vi "VerifConnection.vi"(8 "error in (no error)":errorcluster, 9 "timeout in ms (1000)":u32=1000, 10 "device connected in":bool, 11 "Server in":refnum<class "Server.lvclass">) -> (0 "error out":errorcluster, 3 "Server out":refnum<class "Server.lvclass">)   [LabVIEW 2018, in "Server.lvclass"]
uses:
  Server.lvclass
  Server.lvclass/Server.ctl
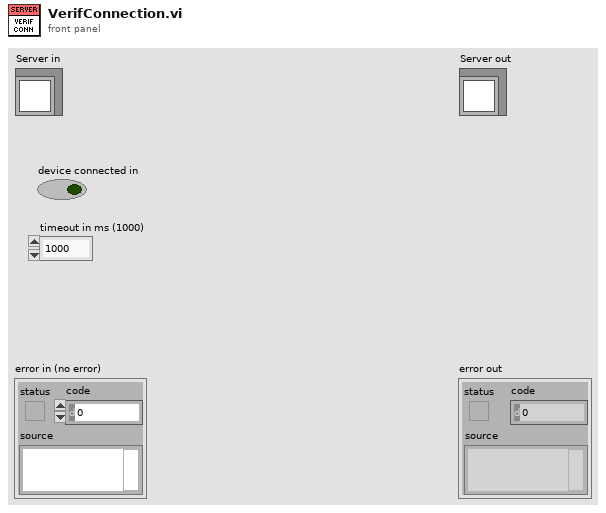
[diagram p1: front panel]
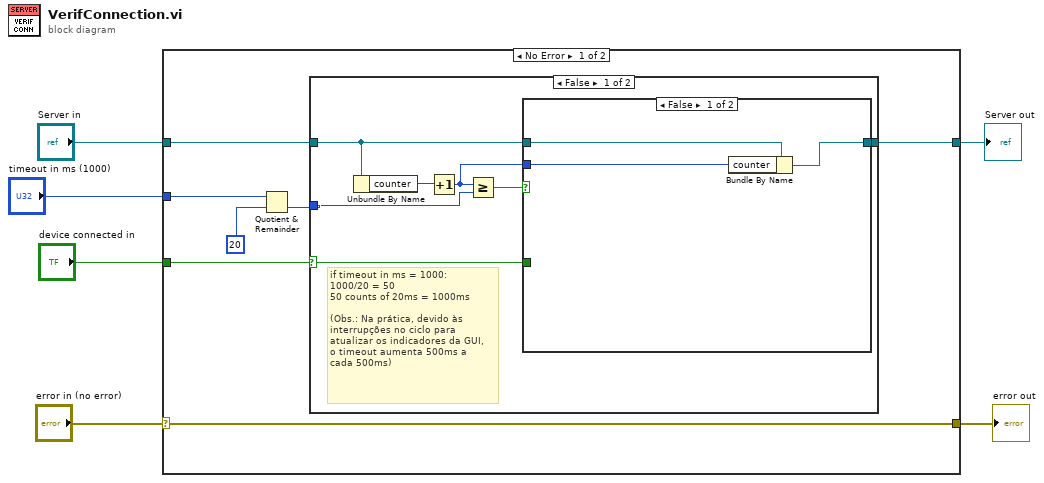
[diagram p0: block diagram]
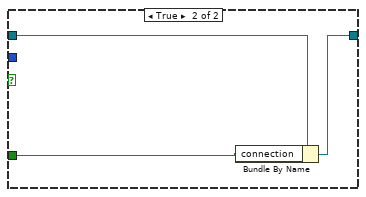
[diagram p2: hidden frame]
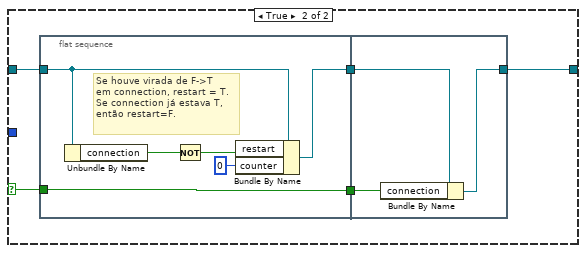
[diagram p3: hidden frame]
diagram:
  n1 = case shown="No Error" "error in (no error)" {
    selector: "error in (no error)" -> [w10 w42]
    tunnel: [w10 w42] -> w5
    tunnel: [w11 w41] -> w3
    tunnel: "Server in" -> [w13 w41]
    tunnel: "device connected in" -> [w12 _]
    tunnel: "timeout in ms (1000)" -> [w9 _]
    frame No Error {
      n2 = Quotient & Remainder(x=w9, y=u32 20) -> (floor(x/y)=w7:u32)  [unwired: 1 out]
      n3 = case shown="False" w12 {
        selector: w12 -> [w17 w29]
        tunnel: w13 -> [w19 w31]
        tunnel: [w16 w27] -> w11
        tunnel: w7 -> [w14 _]
        frame False {
          # "if timeout in ms = 1000:\n1000/20 = 50\n50 counts of 20ms = 1000ms\n\n(Obs.: Na prática, devido às\ninterrupções no ciclo para \natualizar os indicadores da GUI, \no timeout aumenta 500ms a \ncada 500ms)"
          n4 = Unbundle By Name(w19) -> ("counter"=w20:u32)
          n5 = Increment(x=w20) -> (x+1=w15:u32)
          n6 = Greater Or Equal?(x=w15, y=w14) -> (x >= y?=w18:bool)
          n7 = case shown="False" w18 {
            tunnel: w19 -> [w23 w24]
            tunnel: w17 -> [_ w26]
            tunnel: [w22 w25] -> w16
            tunnel: w15 -> [w21 _]
            frame False {
              n8 = Bundle By Name(cluster=w23, "counter"=w21) -> (w22:refnum<class "Server.lvclass">)
            }
            frame True {
              n9 = Bundle By Name(cluster=w24, "connection"=w26) -> (w25:refnum<class "Server.lvclass">)
            }
          }
        }
        frame True {
          n10 = flat-sequence {
            tunnel: w31 -> [w37]
            tunnel: [w34] -> w30
            tunnel: w29 -> [w32]
            tunnel: [w32] -> w28
            tunnel: w30 -> [w40]
            tunnel: w28 -> [w39]
            tunnel: [w38] -> w27
            frame #0 {
              # "Se houve virada de F->T\nem connection, restart = T.\nSe connection já estava T,\nentão restart=F."
              n11 = Unbundle By Name(w37) -> ("connection"=w36:bool)
              n12 = Not(x=w36) -> (.not. x?=w35:bool)
              n13 = Bundle By Name(cluster=w37, "restart"=w35, "counter"=u32 0) -> (w34:refnum<class "Server.lvclass">)
            }
            frame #1 {
              n14 = Bundle By Name(cluster=w40, "connection"=w39) -> (w38:refnum<class "Server.lvclass">)
            }
          }
        }
      }
    }
    frame Error {
    }
  }
  "error out" <- w5
  "Server out" <- w3
